vi "Flash Device.vi"(8 "error in":errorcluster, 11 "MPLab in":refnum<class "MPLab.lvclass">) -> (0 "error out":errorcluster, 3 "MPLab out":refnum<class "MPLab.lvclass">)   [LabVIEW 2018, in "MPLab.lvlib" / "MPLab.lvclass"]
uses:
  MPLab.lvclass
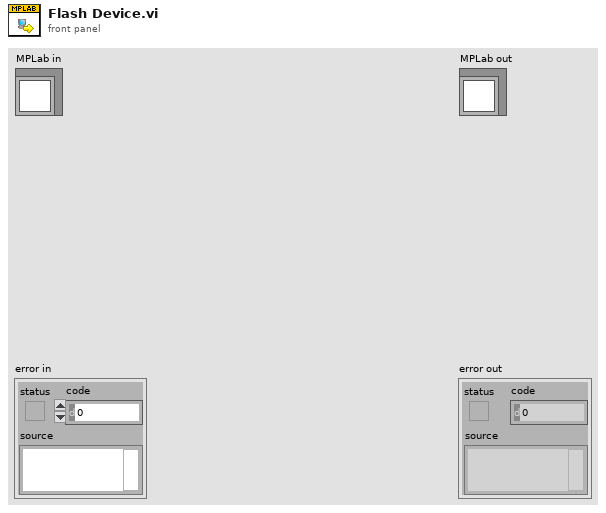
[diagram p1: front panel]
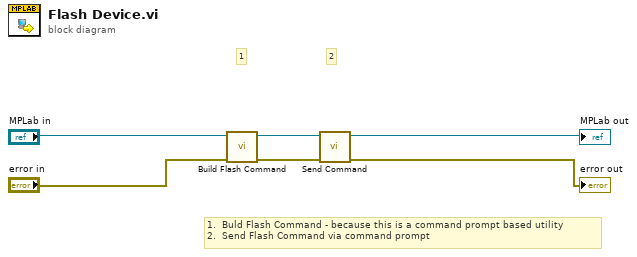
[diagram p0: block diagram]
diagram:
  # "1.  Buld Flash Command - because this is a command prompt based utility\n2.  Send Flash Command via command prompt"
  # "2"
  # "1"
  n1 = call "Build Flash Command.vi"("error in"="error in", "MPLab in"="MPLab in") -> ("error out"=w4:errorcluster, "MPLab out"=w3:refnum<class "MPLab.lvclass">)  [unwired: 8 in]
  n2 = call "Send Command.vi"("error in"=w4, "MPLab in"=w3) -> ("error out"=→"error out":errorcluster, "MPLab out"=→"MPLab out":refnum<class "MPLab.lvclass">)  [unwired: 8 in]
